vi "data_aquisition_spec_pressure.vi"() -> ()   [LabVIEW 2011]
panel:
  in  "Shot Number":i32=120326201
  in  "Take Data w/o Event":bool
  in  "Integration Times (ms)":i32[](array[numeric])
  in  "Spec. Comments":string="no comments"
  out "Shot Progress":u8(slide) scale=0.0..100.0
  in  "Lens and Fiber":string="50mm, P1000-2-UV/VIS EOS00019, 727-733-2447"
  in  "Pressure MDSPlus":bool=TRUE
  in  "Spec. Store":bool=TRUE
  in  "Angle 2":dbl=157.5
  in  "Z 2":dbl=1.0
  in  "Radius 2":dbl
  in  "Z 1":dbl=-1.0
  in  "Angle 1":dbl=157.5
  in  "Radius 1":dbl
  out "Total Counts":cluster{"Y":dbl[], "Y":dbl[]}[](graph)
  out "Pressure Output":cluster{"Y":dbl[], "Y":dbl[]}[](graph)
  in  "Spec. Data":bool=TRUE
  in  "Pressure Data":bool=TRUE
  in  "Sample Rate (1/s)":dbl=10.0
  in  "Backup File Directory":path=path "Z:/usb650_d_tmp_data"
  in  "Maximum #":i32=100
  in  "Delay (s)":dbl
  in  "stop":bool caption="Please use stop button to end program!"
  in  "Tree":string="machine"
  in  "Start Event":string="Shot_Init"
  in  "MDSPlus Host":string="shanghai.ph.utexas.edu"
  out "MDSPlus Connect Status":i32
  out "Shot Number Recorded":i32
  in  "Begin wait for next shot event":bool
  out "Spectrometer Detected":bool
  in  "Length of Shot (s)":dbl=30.0
  # "Fields can be changed in between mds events before pressing the \"wait\" button.\n\nProgram will then wait for mds event and then take data. Wait button must be pressed for each shot."
  # "Shot Event"
  # "Spectroscopic Settings"
  # "Integration Path"
  # "Ion Guage Settings"
  # "MDSPlus Settings"
  # "Backup File Settings"
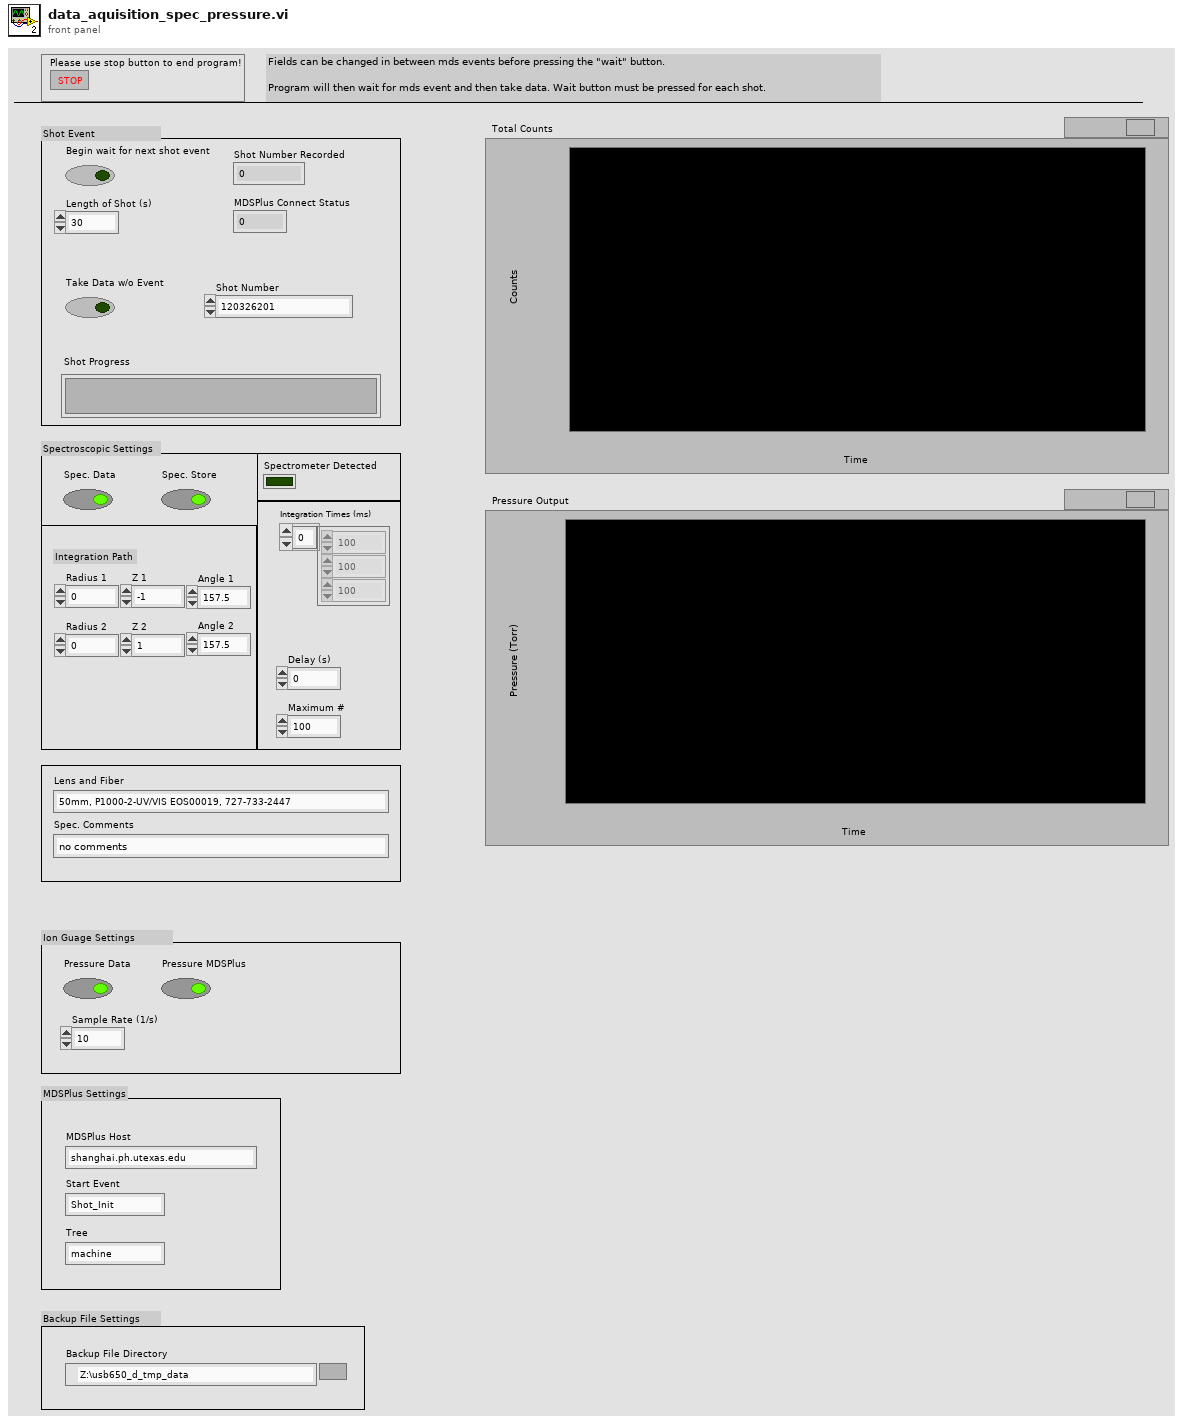
[diagram p1: front panel]
types:
  T1 = enum16{"open", "replace", "create", "open or create", "replace or create", "replace or create with confirmation"}
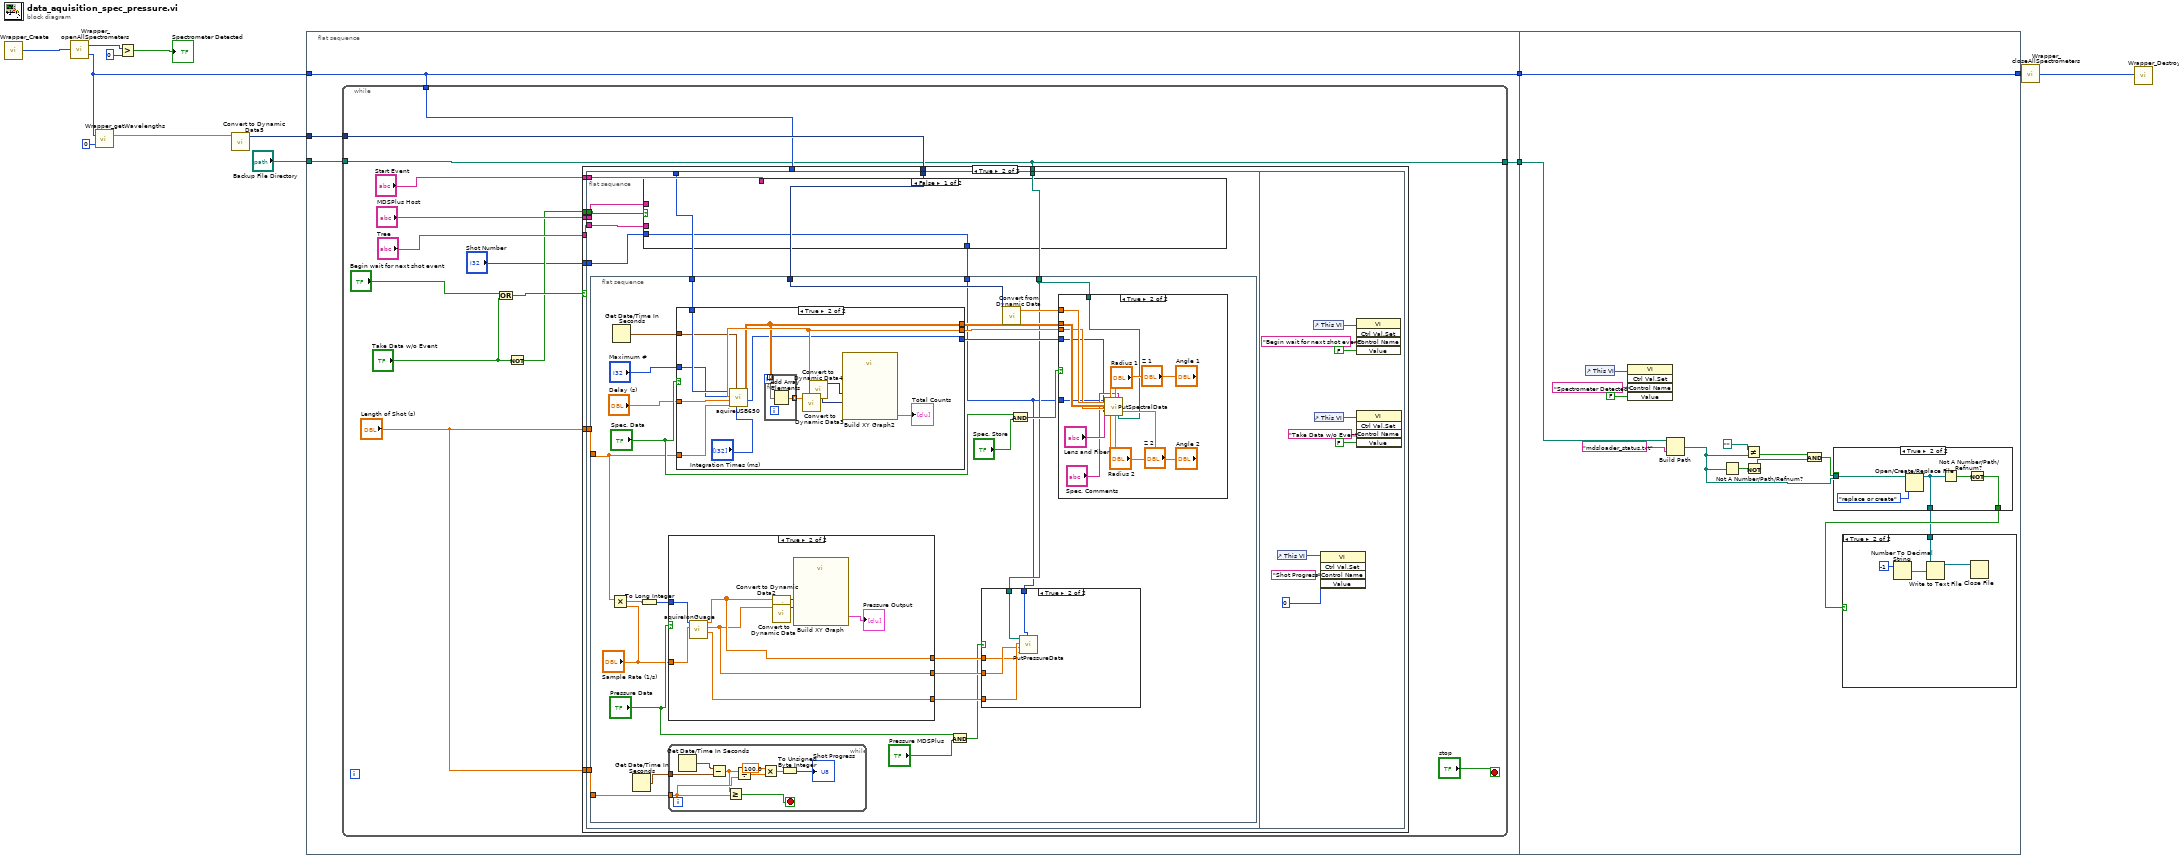
[diagram p0: block diagram]
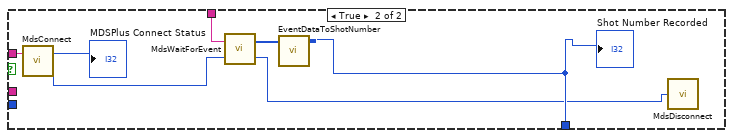
[diagram p3: hidden frame]
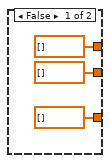
[diagram p4: hidden frame]
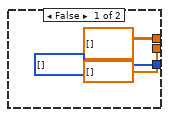
[diagram p5: hidden frame]
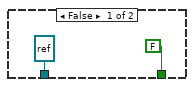
[diagram p9: hidden frame]
diagram:
  n1 = call "Wrapper_Create.vi"() -> ("Wrapper"=w13:u32)
  n2 = call "Wrapper_openAllSpectrometers.vi"("Wrapper In"=w13) -> ("Number of Spectrometers"=w11:i32, "Wrapper Out"=w8:u32)
  n3 = call "Wrapper_getWavelengths.vi"("Index"=0, "Wrapper"=w8) -> ("WL Values"=w4:dbl[])  [unwired: 1 out]
  n4 = Greater?(x=w11, y=0) -> (0:→"Spectrometer Detected":bool)
  n5 = call "Convert to Dynamic Data5"("Array"=w4) -> ("Dynamic Data Type"=w3:dynamicdata)  [unwired: 3 in]
  n6 = flat-sequence {
    tunnel: w8 -> [w17]
    tunnel: [w17] -> w5
    tunnel: w3 -> [w16]
    tunnel: "Backup File Directory" -> [w15]
    tunnel: [w14] -> w1
    tunnel: [w165] -> w7
    tunnel: w5 -> [w165]
    tunnel: w1 -> [w152]
    frame #0 {
      n7 = while {
        tunnel: w17 -> [w24]
        tunnel: w16 -> [w26]
        tunnel: w15 -> [w19]
        tunnel: [w19] -> w14
        stop <- "stop" stop-if-true
        n8 = Or(x="Begin wait for next shot event", y="Take Data w/o Event") -> (x .or. y?=w23:bool)
        n9 = Not(x="Take Data w/o Event") -> (.not. x?=w20:bool)
        n10 = case shown="True" w23 {
          tunnel: "Start Event" -> [_ w40]
          tunnel: "Tree" -> [_ w38]
          tunnel: "MDSPlus Host" -> [_ w39]
          tunnel: "Length of Shot (s)" -> [_ w37]
          tunnel: w24 -> [_ w36]
          tunnel: w26 -> [_ w35]
          tunnel: w19 -> [_ w34]
          tunnel: "Length of Shot (s)" -> [_ w33]
          tunnel: w20 -> [_ w32]
          tunnel: "Shot Number" -> [_ w31]
          frame False {
          }
          frame True {
            n11 = flat-sequence {
              tunnel: w40 -> [w51]
              tunnel: w39 -> [w50]
              tunnel: w38 -> [w49]
              tunnel: w37 -> [w48]
              tunnel: w36 -> [w47]
              tunnel: w35 -> [w46]
              tunnel: w34 -> [w44]
              tunnel: w33 -> [w45]
              tunnel: w32 -> [w43]
              tunnel: w31 -> [w41]
              frame #0 {
                n12 = flat-sequence {
                  tunnel: w48 -> [w65]
                  tunnel: w47 -> [w76]
                  tunnel: w46 -> [w85]
                  tunnel: w44 -> [w61]
                  tunnel: w45 -> [w82]
                  tunnel: w42 -> [w60]
                  frame #0 {
                    n13 = Multiply(x=w65, y="Sample Rate (1/s)") -> (x*y=w68:dbl)
                    n14 = Get Date/Time In Seconds() -> (seconds since 1Jan1904=w63:timestamp)
                    n15 = Get Date/Time In Seconds() -> (seconds since 1Jan1904=w83:timestamp)
                    n16 = To Long Integer(number=w68) -> (32bit integer=w67:i32)
                    n17 = while {
                      tunnel: w83 -> [w122]
                      tunnel: w82 -> [w120]
                      stop <- w121 stop-if-true
                      n18 = Get Date/Time In Seconds() -> (seconds since 1Jan1904=w123:timestamp)
                      n19 = Subtract(x=w123, y=w122) -> (x-y=w119:dbl)
                      n20 = Greater Or Equal?(x=w119, y=w120) -> (x >= y?=w121:bool)
                      n21 = Divide(x=w119, y=w120) -> (x/y=w118:dbl)
                      n22 = Multiply(x=100.0, y=w118) -> (x*y=w115:dbl)
                      n23 = To Unsigned Byte Integer(number=w115) -> (unsigned 8bit integer=→"Shot Progress":u8)
                    }
                    n24 = case shown="True" "Pressure Data" {
                      tunnel: [dbl[] [] ("Time") w93] -> w81
                      tunnel: [dbl[] [] ("Pressure") w92] -> w80
                      tunnel: [dbl[] [] ("Voltage") w91] -> w79
                      tunnel: "Sample Rate (1/s)" -> [_ w90]
                      tunnel: w67 -> [_ w89]
                      frame False {
                      }
                      frame True {
                        n25 = call "aquireIonGuage.vi"("Sample Rate (1/s)"=w90, "Number of Samples"=w89) -> ("Voltage"=w91:dbl[], "Pressure"=w92:dbl[], "Time"=w93:dbl[])  [unwired: 7 in]
                        n26 = call "Convert to Dynamic Data2"("Array"=w93) -> ("Dynamic Data Type"=w94:dynamicdata)  [unwired: 3 in]
                        n27 = call "Convert to Dynamic Data"("Array"=w92) -> ("Dynamic Data Type"=w95:dynamicdata)  [unwired: 3 in]
                        n28 = call "Build XY Graph"("Y Input"=w95, "X Input"=w94) -> ("XY Graph"=→"Pressure Output":cluster{"Y":dbl[], "Y":dbl[]}[])  [unwired: 3 in, 6 out]
                      }
                    }
                    n29 = case shown="True" "Spec. Data" {
                      tunnel: [dbl[] [] ("Time") w108] -> w78
                      tunnel: [dbl[][] [] ("Spectrum Values") w107] -> w77
                      tunnel: w65 -> [_ w106]
                      tunnel: w76 -> [_ w105]
                      tunnel: "Delay (s)" -> [_ w104]
                      tunnel: "Maximum #" -> [_ w103]
                      tunnel: w63 -> [_ w101]
                      tunnel: [i32[] [] ("Integration Times Out") w100] -> w62
                      frame False {
                      }
                      frame True {
                        n30 = call "aquireUSB650.vi"("Integration Times In"="Integration Times (ms)", "Reference Time"=w101, "Length of Shot (s)"=w106, "Delay Between Integrations (s)"=w104, "Maximum Number of Integrations"=w103, "Wrapper In"=w105) -> ("Integration Times Out"=w100:i32[], "Time"=w108:dbl[], "Spectrum Values"=w107:dbl[][])  [unwired: 3 in]
                        n31 = for {
                          tunnel: w107 -> [w114] mode=indexing
                          tunnel: [w113] -> w112 mode=indexing
                          n32 = Add Array Elements(numeric array=w114) -> (sum=w113:dbl)
                        }
                        n33 = call "Convert to Dynamic Data3"("Array"=w112) -> ("Dynamic Data Type"=w110:dynamicdata)  [unwired: 3 in]
                        n34 = call "Convert to Dynamic Data4"("Array"=w108) -> ("Dynamic Data Type"=w109:dynamicdata)  [unwired: 3 in]
                        n35 = call "Build XY Graph2"("Y Input"=w110, "X Input"=w109) -> ("XY Graph"=→"Total Counts":cluster{"Y":dbl[], "Y":dbl[]}[])  [unwired: 3 in, 6 out]
                      }
                    }
                    n36 = And(x="Pressure Data", y="Pressure MDSPlus") -> (x .and. y?=w72:bool)
                    n37 = case shown="True" w72 {
                      tunnel: w79 -> [_ w142]
                      tunnel: w80 -> [_ w141]
                      tunnel: w81 -> [_ w140]
                      tunnel: w61 -> [_ w139]
                      tunnel: w60 -> [_ w138]
                      frame False {
                      }
                      frame True {
                        n38 = call "PutPressureData.vi"("shot"=w138, "Time"=w140, "Pressure"=w141, "Voltage"=w142, "backup_directory"=w139) -> ()  [unwired: 7 in]
                      }
                    }
                    n39 = call "Convert from Dynamic Data"("Dynamic Data Type"=w85) -> ("Array"=w84:dbl[])  [unwired: 3 in]
                    n40 = And(x="Spec. Data", y="Spec. Store") -> (x .and. y?=w74:bool)
                    n41 = case shown="True" w74 {
                      tunnel: w61 -> [_ w126]
                      tunnel: w77 -> [_ w136]
                      tunnel: w78 -> [_ w135]
                      tunnel: w84 -> [_ w137]
                      tunnel: w62 -> [_ w125]
                      tunnel: w60 -> [_ w124]
                      frame False {
                      }
                      frame True {
                        n42 = call "PutSpectralData.vi"("shot"=w124, "wavelengths"=w137, "Counts"=w136, "time"=w135, "Integration Times"=w125, "LensFiber"="Lens and Fiber", "Radius 1"="Radius 1", "Radius 2"="Radius 2", "Z 1"="Z 1", "Z 2"="Z 2", "Angle 1"="Angle 1", "Angle 2"="Angle 2", "Comments"="Spec. Comments", "backup_directory"=w126) -> ()  [unwired: 6 in]
                      }
                    }
                  }
                }
                n43 = case shown="False" w43 {
                  tunnel: w51 -> [_ w58]
                  tunnel: w50 -> [_ w56]
                  tunnel: w49 -> [_ _]
                  tunnel: [w52 w54] -> w42
                  tunnel: w41 -> [w52 _]
                  frame False {
                  }
                  frame True {
                    n44 = call "MdsConnect.vi"("Host"=w56) -> ("FlowControlOut"=w55:i32, "Status"=→"MDSPlus Connect Status":i32)  [unwired: 1 in]
                    n45 = call "MdsWaitForEvent.vi"("FlowControlIn"=w55, "Event"=w58) -> ("FlowControlOut"=w53:i32, "EventData"=w59:u8[])
                    n46 = call "EventDataToShotNumber.vi"("EventDataIn"=w59) -> ("ShotNumberOut"=w54:i32)  [unwired: 10 in]
                    "Shot Number Recorded" <- w54
                    n47 = call "MdsDisconnect.vi"("FlowControlIn"=w53) -> ()  [unwired: 1 out]
                  }
                }
              }
              frame #1 {
                n48 = control-ref of="This VI"() -> (w148:refnum<vi>)
                n49 = control-ref of="This VI"() -> (w151:refnum<vi>)
                n50 = control-ref of="This VI"() -> (w145:refnum<vi>)
                n51 = invoke class="VI" method="Ctrl Val.Set"(reference=w148, "Control Name"="Shot Progress", "Value"=0) -> ()  [unwired: 2 in, 5 out]
                n52 = invoke class="VI" method="Ctrl Val.Set"(reference=w151, "Control Name"="Begin wait for next shot event", "Value"=FALSE) -> ()  [unwired: 2 in, 5 out]
                n53 = invoke class="VI" method="Ctrl Val.Set"(reference=w145, "Control Name"="Take Data w/o Event", "Value"=FALSE) -> ()  [unwired: 2 in, 5 out]
              }
            }
          }
        }
      }
    }
    frame #1 {
      n54 = control-ref of="This VI"() -> (w164:refnum<vi>)
      n55 = invoke class="VI" method="Ctrl Val.Set"(reference=w164, "Control Name"="Spectrometer Detected", "Value"=FALSE) -> ()  [unwired: 2 in, 5 out]
      n56 = Build Path(base path=w152, name or relative path="mdsloader_status.txt") -> (appended path=w153:path)
      n57 = Not A Number/Path/Refnum?(number/path/refnum=w153) -> (NaN/Path/Refnum?=w161:bool)
      n58 = Not Equal?(x=path "", y=w153) -> (x != y?=w160:bool)
      n59 = Not(x=w161) -> (.not. x?=w159:bool)
      n60 = And(x=w160, y=w159) -> (x .and. y?=w158:bool)
      n61 = case shown="True" w158 {
        tunnel: [FALSE w174] -> w157
        tunnel: [refnum<file> refnum ("refnum out") w173] -> w156
        tunnel: w153 -> [_ w172]
        frame False {
        }
        frame True {
          n62 = Open/Create/Replace File(file path (use dialog)=w172, operation (0:open)=T1."replace or create") -> (refnum out=w173:refnum<file>)  [unwired: 4 in, 2 out]
          n63 = Not A Number/Path/Refnum?(number/path/refnum=w173) -> (NaN/Path/Refnum?=w175:bool)
          n64 = Not(x=w175) -> (.not. x?=w174:bool)
        }
      }
      n65 = case shown="True" w157 {
        tunnel: w156 -> [_ w169]
        frame False {
        }
        frame True {
          n66 = Number To Decimal String(number=-1) -> (decimal integer string=w167:string)  [unwired: 1 in]
          n67 = Write to Text File(file (use dialog)=w169, text=w167) -> (refnum out=w168:refnum<file>)  [unwired: 2 in, 2 out]
          n68 = Close File(refnum=w168) -> ()  [unwired: 1 in, 2 out]
        }
      }
    }
  }
  n69 = call "Wrapper_closeAllSpectrometers.vi"("Wrapper In"=w7) -> ("Wrapper Out"=w6:u32)
  n70 = call "Wrapper_Destroy.vi"("Wrapper"=w6) -> ()
